vi "Write Data.vi"(8 "error in (no error)":errorcluster, 9 "Publication Time":timestamp, 10 "Value":variant, 11 "ValueReferenceTransport In":refnum<class "ValueReferenceTransport.lvclass">) -> (0 "error out":errorcluster, 3 "ValueReferenceTransport Out":refnum<class "ValueReferenceTransport.lvclass">)   [LabVIEW 2020, in "ValueReferenceTransport.lvclass"]
doc: "<License>\nCopyright © 2017 Composed Systems, LLC | All rights reserved\nwww.composed.io\n\nAuthor: Ethan Stern <ethan.stern@composed.io>\n\nThis software is provided \"AS IS\" WITHOUT WARRANTIES, either express or implied, AND IS FOR EDUCATIONAL PURPOSES ONLY.\n</License>"
uses:
  <vilib>/gpm_packages/@cs/transport/Source/Concrete/ValueReferenceTransport/ValueReferenceTransport.lvclass
  <vilib>/gpm_packages/@cs/transport/Source/Concrete/ValueReferenceTransport/ValueReferenceTransport.lvclass/ValueReferenceTransport.ctl
  <vilib>/Utility/error.llb/Error Cluster From Error Code.vi
  <vilib>/ErrorRing/Error Ring.xnode
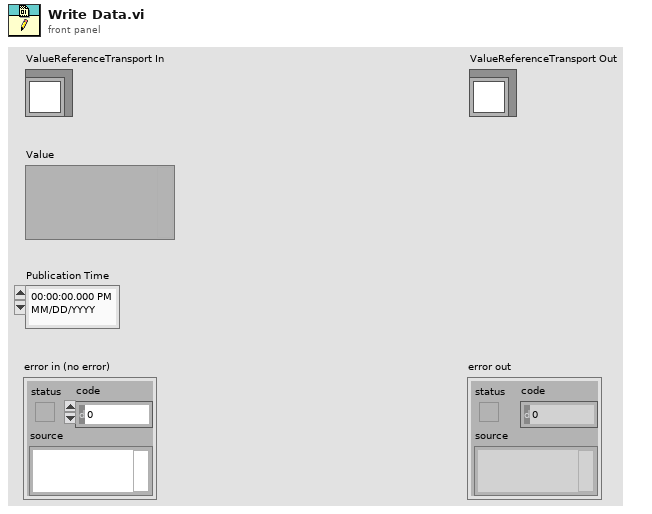
[diagram p1: front panel]
types:
  T1 = cluster{"Data":variant, "Publication Time":timestamp}
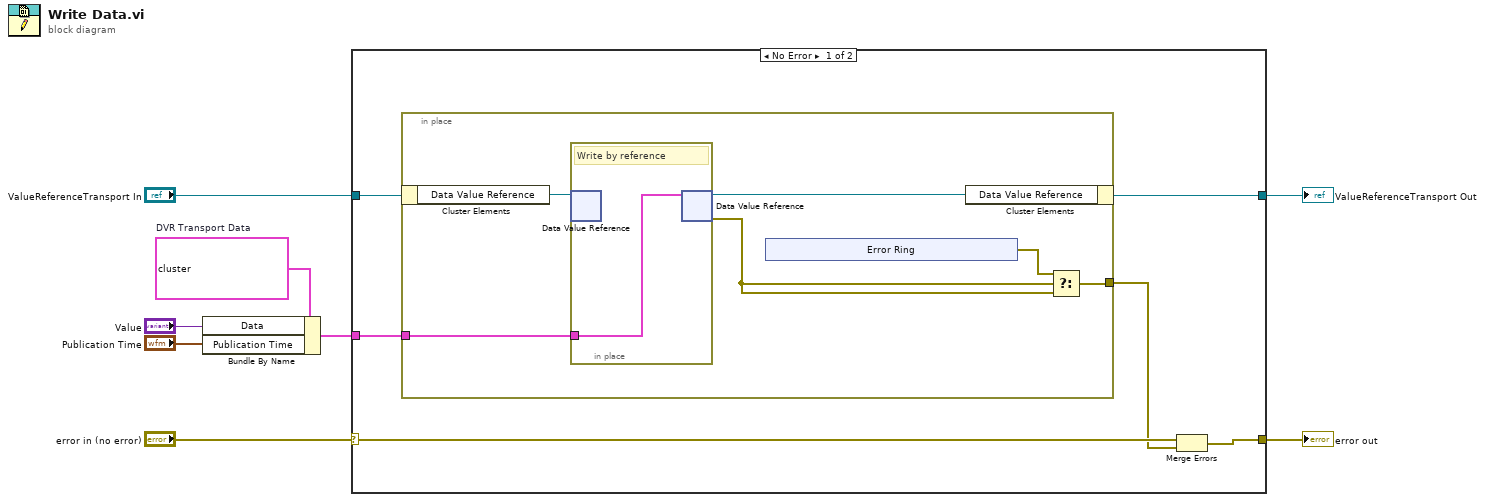
[diagram p0: block diagram]
diagram:
  w6 = T1 {"Data"=variant, "Publication Time"=timestamp(0 s since 1904-01-01)}  # DVR Transport Data
  n1 = Bundle By Name(cluster=w6, "Data"="Value", "Publication Time"="Publication Time") -> (w4:T1)
  n2 = case shown="No Error" "error in (no error)" {
    selector: "error in (no error)" -> [w14 w27]
    tunnel: [w13 w27] -> w7
    tunnel: w4 -> [w11 _]
    tunnel: "ValueReferenceTransport In" -> [w10 w28]
    tunnel: [w9 w28] -> w1
    frame No Error {
      n3 = in-place {
        in-place-border: [w16] -> w12
        in-place-border: w11 -> [w20]
        n4 = in-place-cluster #1(w10) -> ("Data Value Reference"=w19:refnum<data-value>)
        n5 = in-place {
          in-place-border: w20 -> [w21]
          # "Write by reference"
          n6 = in-place-dvr #2(w19) -> ()  [unwired: 2 out]
          n7 = in-place-dvr #2(w21) -> (w18:refnum<data-value>, w17:errorcluster)
        }
        n8 = xnode "Error Ring"() -> ("error out"=w15:errorcluster)
        n9 = in-place-cluster #1("Data Value Reference"=w18) -> (w9:refnum<class "ValueReferenceTransport.lvclass">)
        n10 = Select(t=w15, s=w17, f=w17) -> (s? t:f=w16:errorcluster)
      }
      n11 = Merge Errors(w14, w12) -> (w13:errorcluster)
    }
    frame Error {
      # "Transports do not write on upstream error"
    }
  }
  "error out" <- w7
  "ValueReferenceTransport Out" <- w1
